vi "Get Valid Properties.vi"(8 "error in (no error)":errorcluster, 11 "Tone in":refnum<class "Tone.lvclass">) -> (0 "error out":errorcluster, 2 "Properties":string[](array[string]), 3 "Tone out":refnum<class "Tone.lvclass">)   [LabVIEW 2020, in "Tone.lvclass"]
uses:
  Tone.lvclass
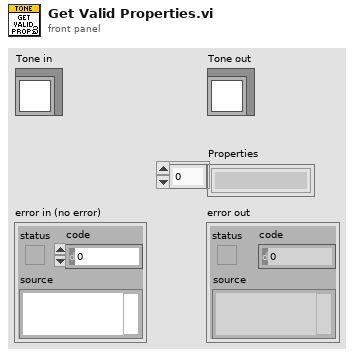
[diagram p1: front panel]
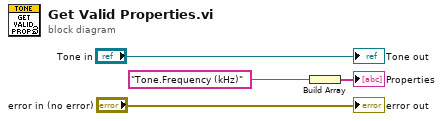
[diagram p0: block diagram]
diagram:
  n1 = Build Array("Tone.Frequency (kHz)" ("String")) -> (→"Properties":string[])
  "error out" <- "error in (no error)"
  "Tone out" <- "Tone in"
